vi "PCA9685_Servo_Control_Example.vi"() -> ()   [LabVIEW 2019]
panel:
  in  "Servo 0°~180° Duty Cycle":dbl(slide) scale=0.02..0.12
  in  "Stop":bool
  in  "Error In":errorcluster
  out "Error Out":errorcluster
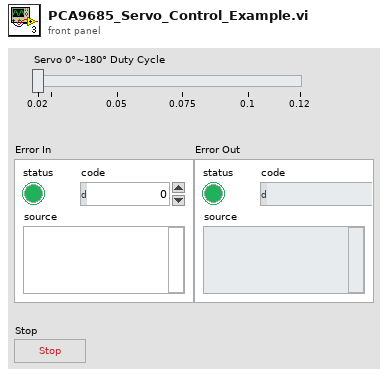
[diagram p1: front panel]
types:
  T1 = enum16{"LED/PWM00", "LED/PWM01", "LED/PWM02", "LED/PWM03", "LED/PWM04", "LED/PWM05", "LED/PWM06", "LED/PWM07", "LED/PWM08", "LED/PWM09", "LED/PWM10", "LED/PWM11", "LED/PWM12", "LED/PWM13", "LED/PWM14", "LED/PWM15"}
  T2 = typedef "I2C.lvlib/I2C Reference.ctl" = cluster{"myRIO Reference":T3, "I2C Channels Enum":T7, "I2C Configuration":T8}
  T3 = typedef "myRIO Generic Hardware Reference.ctl" = cluster{"myRIO Model":T4, "myRIO Hardware Reference":T5}
  T4 = typedef "Hardware Version Enum.ctl" = enum16{"Unknown", "myRIO-1900", "myRIO-1950", "roboRIO", "NI ELVIS RIO CM", "ELVIS III"}
  T5 = typedef "myRIO v1.0 Reference.ctl" = cluster{"Generic FPGA Reference":T6, "Allow multiple opens":bool}
  T6 = typedef "Generic FPGA Reference.ctl" = refnum<k20>
  T7 = typedef "I2C Channels Enum.ctl" = enum16{"Not Connected", "A/I2C", "B/I2C", "I2C/I2C"}
  T8 = typedef "I2C.lvlib/I2C Configuration.ctl" = cluster{"I2C Transfer Rate":T9}
  T9 = typedef "I2C.lvlib/I2C Transfer Rate.ctl" = enum16{"Standard mode (100 kbps)", "Fast mode (400 kbps)"}
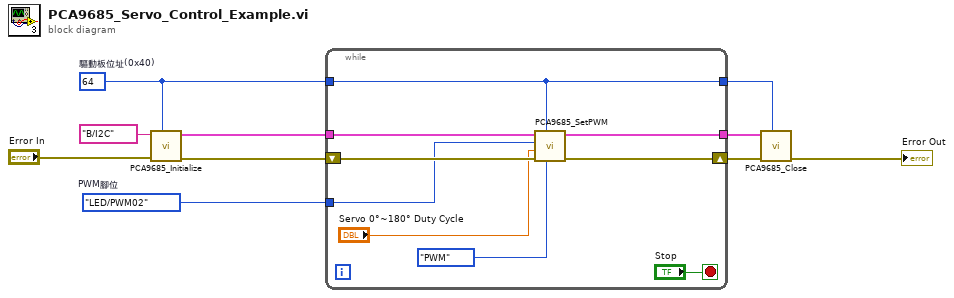
[diagram p0: block diagram]
diagram:
  w1 = T1."LED/PWM02"  # PWM腳位
  w7 = u8 64  # 驅動板位址(0x40)
  n1 = call "PCA9685_Initialize.vi"("驅動板位址(0x40)"=w7, "Error In"="Error In", "I2C腳位"=tag "B/I2C") -> ("Error Out"=w9:errorcluster, "I2C Ref Out"=w10:T2)  [unwired: 7 in]
  n2 = while {
    tunnel: w10 -> [w19]
    tunnel: w7 -> [w12]
    shift-right: [w14] -> w5
    shift-left: w9 -> [w18]
    tunnel: [w13] -> w3
    tunnel: [w12] -> w2
    tunnel: w1 -> [w11]
    stop <- "Stop" stop-if-true
    n3 = call "PCA9685_SetPWM.vi"("控制模式"=enum16{"PWM", "LED ON", "LED OFF"}."PWM", "驅動板位址(0x40)"=w12, "Error In"=w18, "Duty Cycle(0~1)"="Servo 0°~180° Duty Cycle", "PWM腳位"=w11, "I2C Ref In"=w19) -> ("Error Out"=w14:errorcluster, "I2C Ref Out"=w13:T2)  [unwired: 4 in]
  }
  n4 = call "PCA9685_Close.vi"("驅動板位址(0x40)"=w2, "Error In"=w5, "I2C Ref In"=w3) -> ("Error Out"=→"Error Out":errorcluster)  [unwired: 8 in]
